vi "Test Get ATM Message when Depositing.vi"(8 "error in (no error)":errorcluster, 11 "Test Case In":refnum<class "Controller Test.lvclass">) -> (0 "error out":errorcluster, 3 "Test Case Out":refnum<class "Controller Test.lvclass">)   [LabVIEW 2020, in "Controller Test.lvclass"]
uses:
  Controller Test/Controller Test.lvclass
  Controller Test/Controller Test.lvclass/Controller Test.ctl
  01074fa8-ee8a-411d-bc8b-fc92c4f90959.vi
  ATM Controller/ATM Controller.lvclass
  ATM Controller/State.ctl
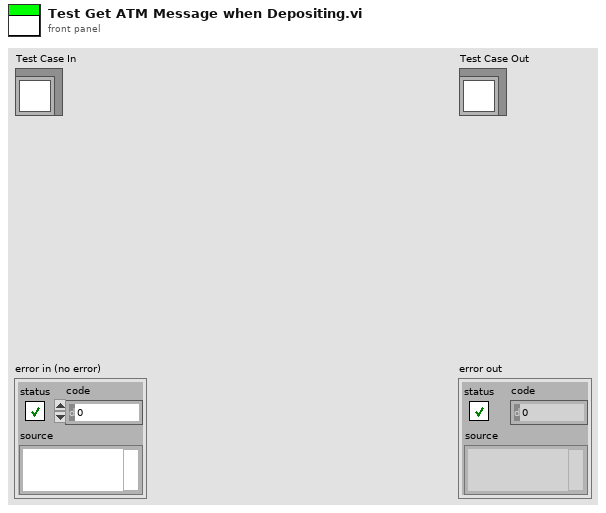
[diagram p1: front panel]
types:
  T1 = typedef "ATM Controller.lvclass/State.ctl" = enum16{"Start", "Card Inserted", "Verification Failed", "Verification Succeeded", "Depositing", "Terminate"}
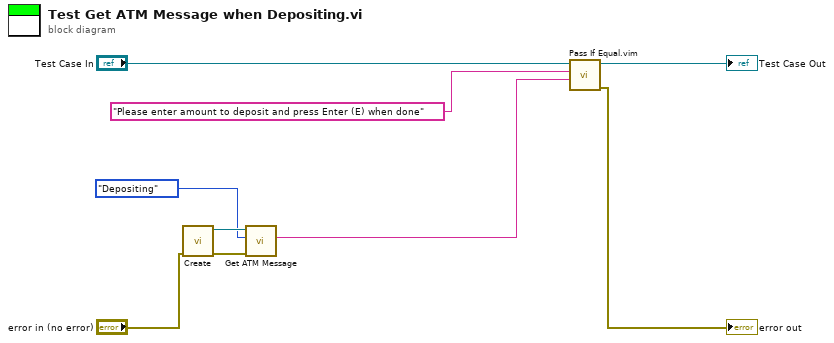
[diagram p0: block diagram]
diagram:
  n1 = call "Create.vi"("error in (no error)"="error in (no error)") -> ("error out"=w4:errorcluster, "ATM Controller out"=w5:refnum<class "ATM Controller.lvclass">)  [unwired: 9 in]
  n2 = call "Get ATM Message.vi"("error in (no error)"=w4, "ATM State"=State."Depositing", "ATM Controller In"=w5) -> ("Message"=w3:string)  [unwired: 6 in, 2 out]
  n3 = call "Pass If Equal.vim"("Actual"=w3, "Expected"="Please enter amount to deposit and press Enter (E) when done" ("Message"), "LUnit Test Case In"="Test Case In") -> ("error out"=→"error out":errorcluster, "LUnit Test Case Out"=→"Test Case Out":refnum<class "Controller Test.lvclass">)  [unwired: 7 in]
